vi "Transform.vi"(8 "error in (no error)":errorcluster caption="entrée d'erreur (pas d'erreur)", 9 "y":string[][](array[string]), 10 "X":string[][](array[string]), 11 "Nystroem.lvclass":refnum<class "Nystroem.lvclass">) -> (0 "error out":errorcluster caption="sortie d'erreur", 2 "Data":T1, 3 "Nystroem.lvclass":refnum<class "Nystroem.lvclass">)   [LabVIEW 2020, in "Nystroem.lvclass"]
doc: "Apply feature map to X.\n\nComputes an approximate feature map using the kernel between some training points and X.\n\nReturns : \n\n- X_transformed : array, shape=(n_samples, n_components)\nTransformed data."
uses:
  Nystroem.lvclass
  Nystroem.lvclass/Nystroem.ctl
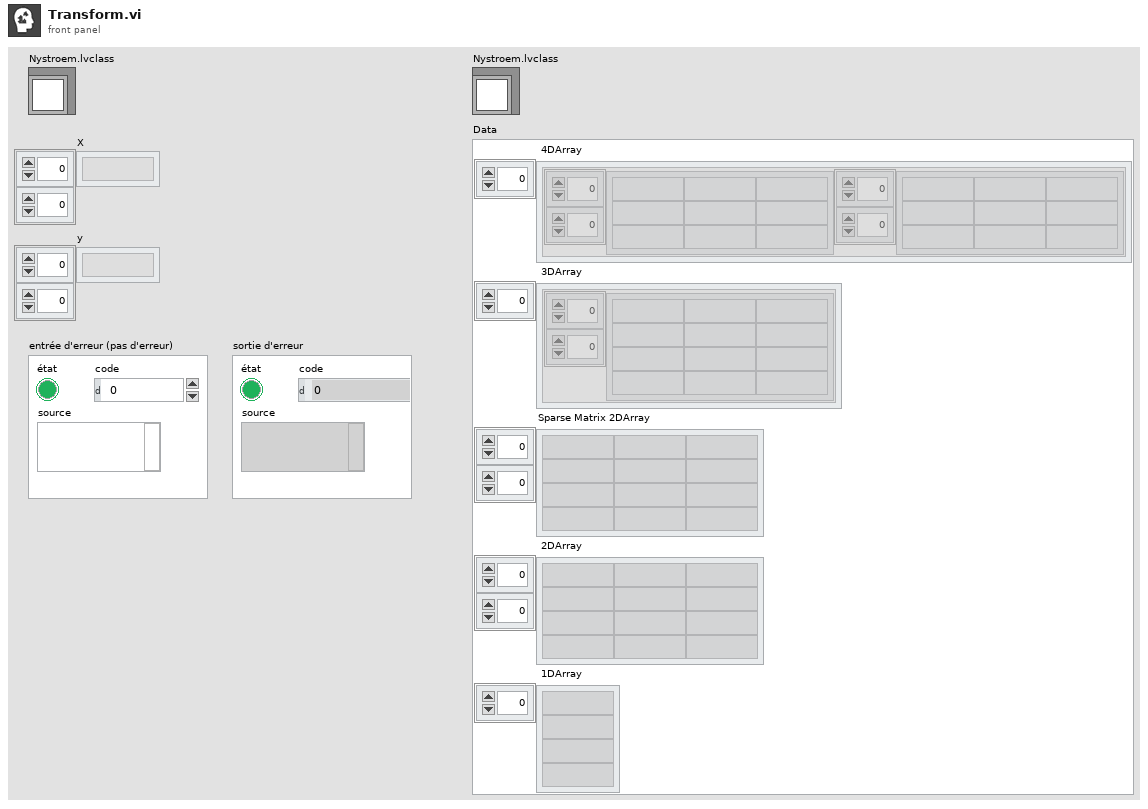
[diagram p1: front panel]
types:
  T1 = cluster{" 4DArray":cluster{"1":string[][], "2":string[][]}[], " 3DArray":cluster{"Tableau":string[][]}[], "Sparse Matrix 2DArray":string[][], " 2DArray":string[][], " 1DArray":string[]}
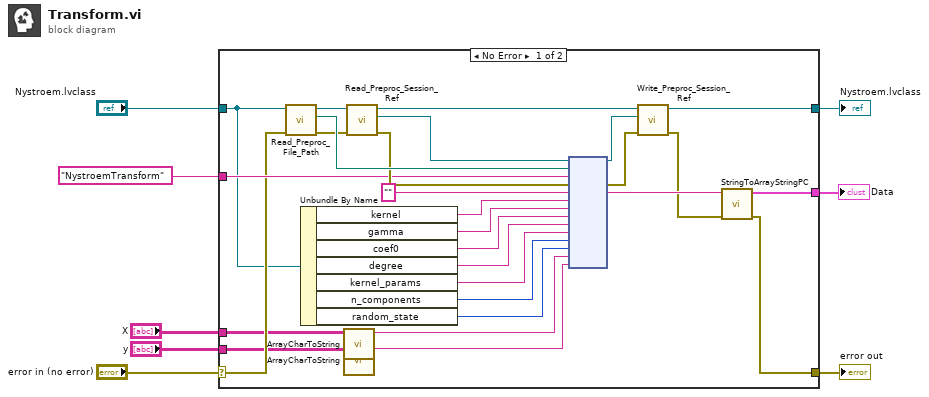
[diagram p0: block diagram]
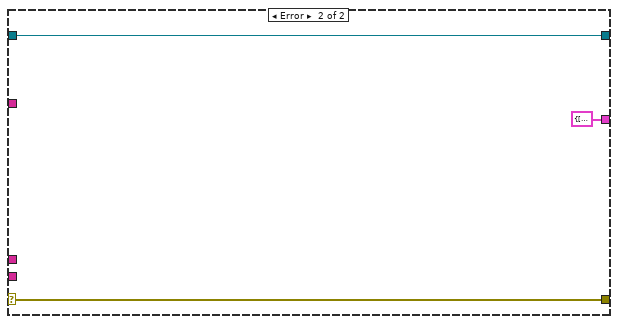
[diagram p2: hidden frame]
diagram:
  n1 = case shown="No Error" "error in (no error)" {
    selector: "error in (no error)" -> [w24 w39]
    tunnel: [w9 w39] -> w7
    tunnel: [w13 w38] -> w5
    tunnel: "Nystroem.lvclass" -> [w23 w38]
    tunnel: "NystroemTransform" ("Fonction") -> [w25 _]
    tunnel: "X" -> [w17 _]
    tunnel: "y" -> [w15 _]
    tunnel: [w11 T1 {" 4DArray"=[], " 3DArray"=[], "Sparse Matrix 2DArray"=[], " 2DArray"=[], " 1DArray"=[]} ("Data")] -> w1
    frame No Error {
      n2 = call-dynamic "Read_Preproc_File_Path.vi"("error in (no error)"=w24, "Python in"=w23) -> ("error out"=w31:errorcluster, "File_Path"=w34:path, "Python out"=w36:refnum<class "Nystroem.lvclass">)  [unwired: 7 in]
      n3 = Unbundle By Name(w23) -> ("kernel"=w27:string, "gamma"=w26:string, "coef0"=w22:string, "degree"=w21:string, "kernel_params"=w20:string, "n_components"=w19:i32, "random_state"=w18:i32)
      n4 = call "ArrayCharToString.vi"("TAB"=w17) -> ("Instruction"=w16:string)  [unwired: 10 in]
      n5 = call "ArrayCharToString.vi"("TAB"=w15) -> ("Instruction"=w14:string)  [unwired: 10 in]
      n6 = call-dynamic "Read_Preproc_Session_Ref.vi"("error in (no error)"=w31, "Python in"=w36) -> ("error out"=w32:errorcluster, "Session_ref"=w33:refnum<k35>, "Python out"=w35:refnum<class "Nystroem.lvclass">)  [unwired: 7 in]
      n7 = node(w33, w34, w25, w32, "", w27, w26, w22, w21, w20, w19, w18, w16, w14) -> (w28:refnum<k35>, w30:errorcluster, w12:string)  [unwired: 9 in, 2 out]
      n8 = call-dynamic "Write_Preproc_Session_Ref.vi"("error in (no error)"=w30, "Session_ref"=w28, "Python in"=w35) -> ("error out"=w10:errorcluster, "Python out"=w13:refnum<class "Nystroem.lvclass">)  [unwired: 7 in]
      n9 = call "StringToArrayStringPC.vi"("sortie d'erreur"=w10, "Return value"=w12) -> ("sortie d'erreur"=w9:errorcluster, "Data"=w11:T1)  [unwired: 8 in]
    }
    frame Error {
    }
  }
  "error out" <- w7
  "Nystroem.lvclass" <- w5
  "Data" <- w1
